vi "DAQ@WaveFormGenerate__Parameter.vi"(1 "ParamterIn":string) -> (0 "ParamterOut":string)   [LabVIEW 2019]
panel:
  in  "ParameterS":string(combo)
  in  "SPS":string(combo)
  in  "WaveFromType":string(combo)
  in  "WaveFormName":string(combo)
  in  "Confirm":bool
  # "DAQ@WaveFormGenerate $WaveForm,$Type,$SPS,$ParameterS...............\n------------------------------------------------------------------------------------------------------------------------------------------\nSQUARE        $WaveFormName,SQUARE,$SPS,$timeinterval,$frequency,$amplitude,$offset,$phase\nSINE             $WaveFormName,SINE,$SPS,$timeinterval,$frequency,$amplitude,$offset,$phase\nTRIANGLE     $WaveFormName,TRIANGLE,$SPS,$timeinterval,$frequency,$amplitude,$offset,$phase\nSAWTOOTH  $WaveFormName,SAWTOOTH,$SPS,$timeinterval,$frequency,$amplitude,$offset,$phase\nSTEP            $WaveFormName,STEP,$SPS,0,Value0,[,Time1,Value1,..............]\nRAMP           $WaveFormName,RAMP,$SPS,0,Value0,[,Time1,Value1,..............]\nPULSE          $WaveFormName,PULSE,$SPS,$LEN,$time0,$value0,$duty0[,$time1,$value1,$duty1¡K¡K¡K.]\nPWM            $WaveFormName,PWM,$SPS,$LEN,$frequency,$amplitude,$offset,$phase,$duty"
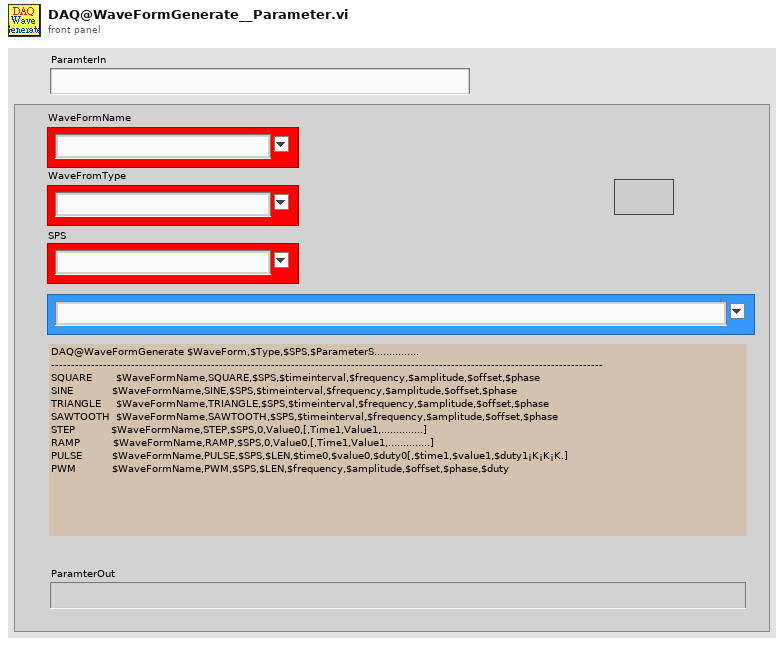
[diagram p1: front panel]
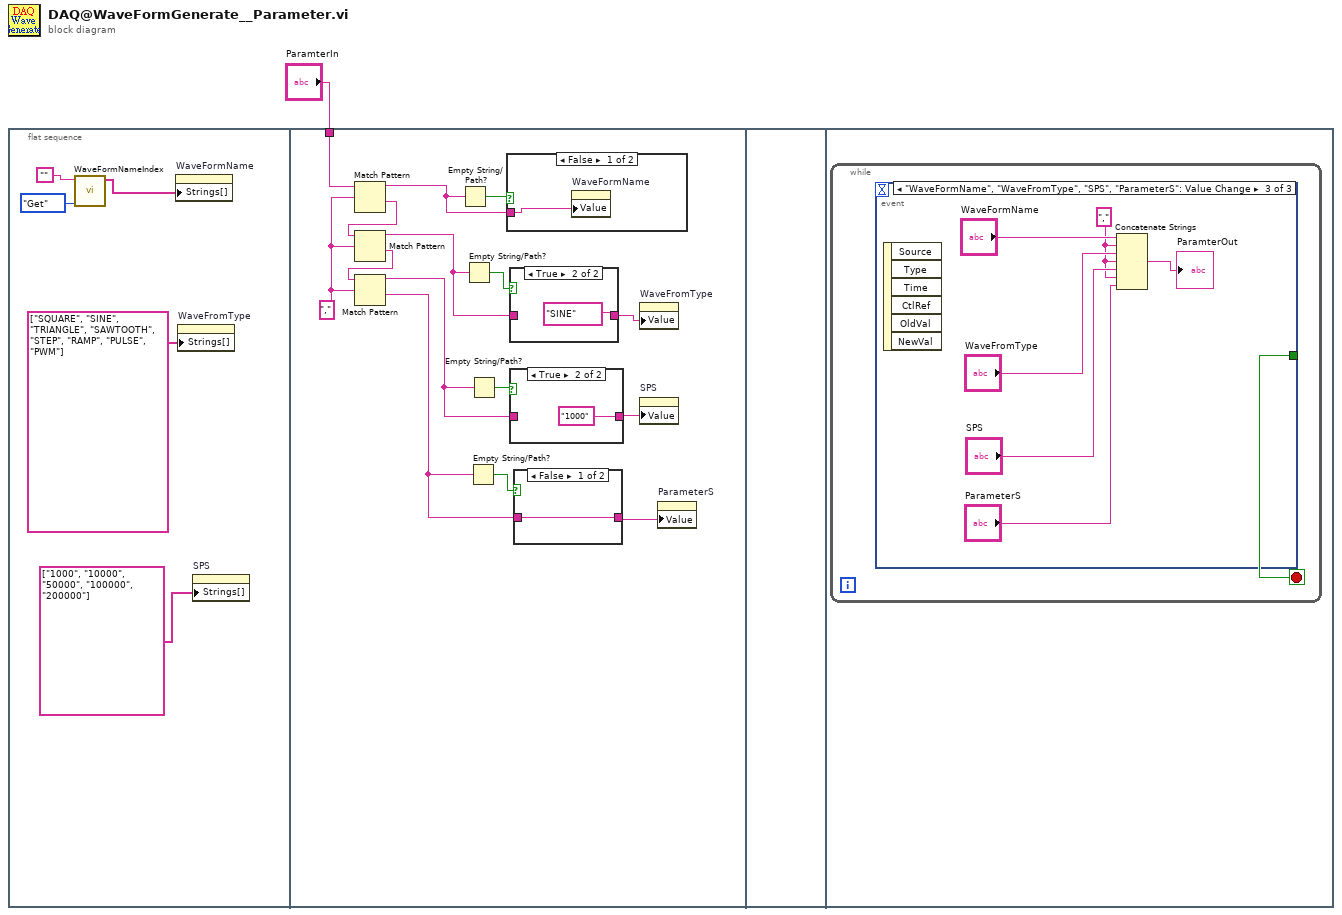
[diagram p0: block diagram]
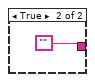
[diagram p2: hidden frame]
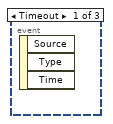
[diagram p6: hidden frame]
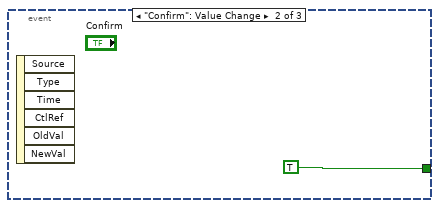
[diagram p7: hidden frame]
diagram:
  n1 = flat-sequence {
    tunnel: "ParamterIn" -> [w14]
    frame #0 {
      n2 = call "WaveFormNameIndex.vi"("OP"=enum16{"Get", "Update", "Init", "GetSPS"}."Get", "WaveFormName"="") -> ("WaveFormNameList"=w3:string[])  [unwired: 6 in, 3 out]
      n3 = property on="WaveFormName" class="CmbBox"("Strings[]"=w3) -> ()  [unwired: 2 in, 2 out]
      n4 = property on="WaveFromType" class="CmbBox"("Strings[]"=string[] ["SQUARE", "SINE", "TRIANGLE", "SAWTOOTH", "STEP", "RAMP", "PULSE", "PWM"] ("Strings []")) -> ()  [unwired: 2 in, 2 out]
      n5 = property on="SPS" class="CmbBox"("Strings[]"=string[] ["1000", "10000", "50000", "100000", "200000"] ("Strings []")) -> ()  [unwired: 2 in, 2 out]
    }
    frame #1 {
      w9 = "," ("search string/char (-)")
      n6 = Match Pattern(string=w14, regular expression=w9) -> (before substring=w13:string, after substring=w12:string)  [unwired: 1 in, 2 out]
      n7 = Match Pattern(string=w12, regular expression=w9) -> (before substring=w11:string, after substring=w10:string)  [unwired: 1 in, 2 out]
      n8 = Match Pattern(string=w10, regular expression=w9) -> (before substring=w8:string, after substring=w7:string)  [unwired: 1 in, 2 out]
      n9 = Empty String/Path?(string/path=w13) -> (empty?=w21:bool)
      n10 = Empty String/Path?(string/path=w11) -> (empty?=w20:bool)
      n11 = Empty String/Path?(string/path=w7) -> (empty?=w16:bool)
      n12 = Empty String/Path?(string/path=w8) -> (empty?=w18:bool)
      n13 = case shown="False" w21 {
        tunnel: w13 -> [w28 _]
        frame False {
          n14 = property on="WaveFormName" class="CmbBox"("Value"=w28) -> ()  [unwired: 2 in, 2 out]
        }
        frame True {
        }
      }
      n15 = case shown="True" w20 {
        tunnel: [w26 "SINE"] -> w19
        tunnel: w11 -> [w26 _]
        frame False {
        }
        frame True {
        }
      }
      n16 = case shown="True" w18 {
        tunnel: [w24 "1000"] -> w17
        tunnel: w8 -> [w24 _]
        frame False {
        }
        frame True {
        }
      }
      n17 = case shown="False" w16 {
        tunnel: [w22 ""] -> w15
        tunnel: w7 -> [w22 _]
        frame False {
        }
        frame True {
        }
      }
      n18 = property on="WaveFromType" class="CmbBox"("Value"=w19) -> ()  [unwired: 2 in, 2 out]
      n19 = property on="SPS" class="CmbBox"("Value"=w17) -> ()  [unwired: 2 in, 2 out]
      n20 = property on="ParameterS" class="CmbBox"("Value"=w15) -> ()  [unwired: 2 in, 2 out]
    }
    frame #2 {
    }
    frame #3 {
      n21 = while {
        stop <- w29 stop-if-true
        n22 = event shown="[2] \"WaveFormName\", \"WaveFromType\", \"SPS\", \"ParameterS\": Value Change" {
          selector: _ -> [_ _ _]
          dyn-events: _ -> [_ _ _]
          timeout: _ -> [_ _ _]
          tunnel: [_ TRUE _] -> w29
          event Timeout {
            n23 = event-data() -> ()  [unwired: 1 in, 3 out]
          }
          event "Confirm": Value Change {
            n24 = event-data() -> ()  [unwired: 1 in, 6 out]
          }
          event "WaveFormName", "WaveFromType", "SPS", "ParameterS": Value Change {
            w32 = ","
            n25 = event-data() -> ()  [unwired: 1 in, 6 out]
            n26 = Concatenate Strings("WaveFormName", w32, "WaveFromType", w32, "SPS", w32, "ParameterS") -> (→"ParamterOut":string)
          }
        }
      }
    }
  }
